vi "push.vi"(0 "push":bool) -> ()   [LabVIEW 2018]
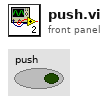
[diagram p1: front panel]
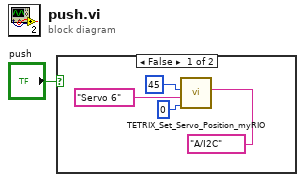
[diagram p0: block diagram]
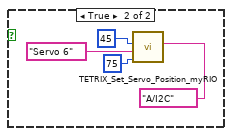
[diagram p2: hidden frame]
diagram:
  n1 = case shown="False" "push" {
    frame False {
      n2 = call <vilib>:"TETRIX_Set_Servo_Position_myRIO.vi"("myRIO MXP Port A/B"=tag "A/I2C", "Set Servo Position (0 - 180 degrees)"=u8 0, "Select Channel"="Servo 6", "Controller ID#  (I2C Address)"=u8 45) -> ()  [unwired: 3 in, 1 out]
    }
    frame True {
      n3 = call <vilib>:"TETRIX_Set_Servo_Position_myRIO.vi"("myRIO MXP Port A/B"=tag "A/I2C", "Set Servo Position (0 - 180 degrees)"=u8 75, "Select Channel"="Servo 6", "Controller ID#  (I2C Address)"=u8 45) -> ()  [unwired: 3 in, 1 out]
    }
  }
